vi "Create Generic IO Profile.vi"(8 "error in":errorcluster, 11 "Cia401Profile in":refnum<class "CiA401 Generic IO Profile.lvclass">) -> (0 "error out":errorcluster, 3 "Cia401Profile out":refnum<class "CiA401 Generic IO Profile.lvclass">)   [LabVIEW 2020, in "CiA401 Generic IO Profile.lvclass"]
uses:
  CiA401 Generic IO Profile.lvclass
  CiA401 Generic IO Profile.lvclass/CiA401 Generic IO Profile.ctl
  D:/git/CANopen-LabVIEW/source/Device Profile/Device Profile.lvclass
  D:/git/CANopen-LabVIEW/Profiles/401 Generic IO/CiA401 Generic IO Profile.lvclass
  source/Device Profile/Device Profile.lvclass
  source/Typedefs/Data Type.ctl
  source/CANopen.lvlib
  source/Typedefs/OD Entry Spec.ctl
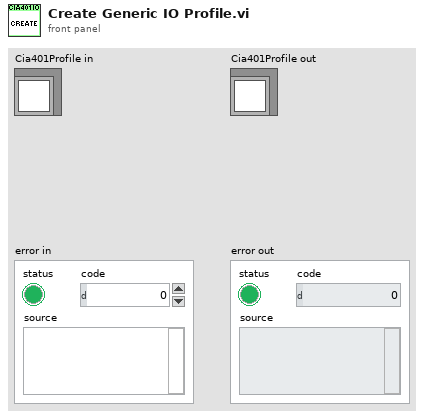
[diagram p1: front panel]
types:
  T1 = typedef "CiA401 Generic IO Profile.lvclass/IO Capabilities.ctl" = cluster{"hasDigitialInputs":bool, "hasDigitalOutputs":bool, "hasAnalogInputs":bool, "hasAnalogOutputs":bool}
  T2 = typedef "CANopen.lvlib/OD Entry Spec.ctl" = cluster{"Index":u16, "Sub Index":u8, "Name":string, "Data Type":T3}
  T3 = typedef "CANopen.lvlib/Data Type.ctl" = u16
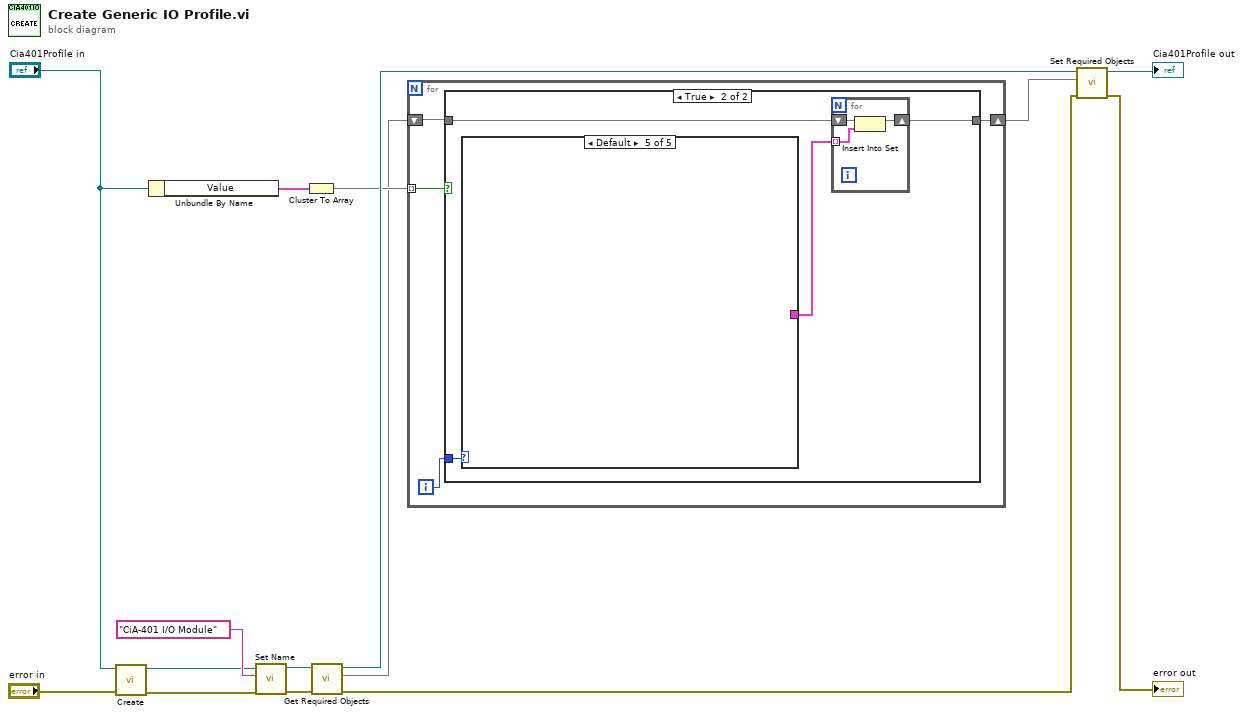
[diagram p0: block diagram]
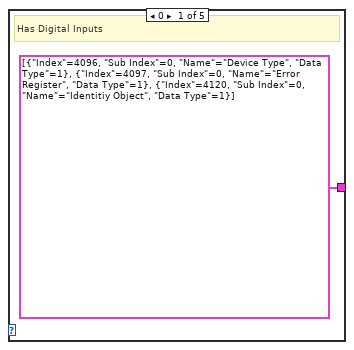
[diagram p3: hidden frame]
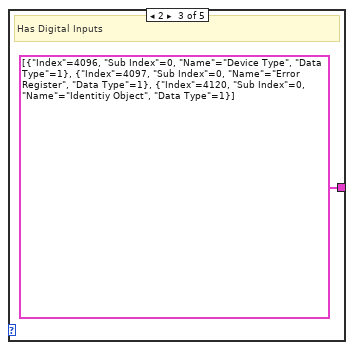
[diagram p5: hidden frame]
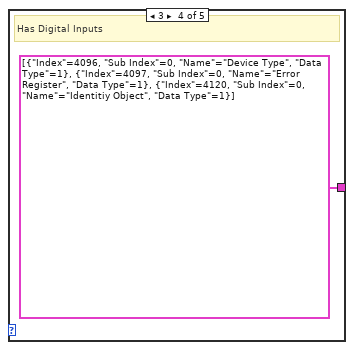
[diagram p6: hidden frame]
diagram:
  n1 = call-dynamic "Create.vi"("error in"="error in", "Device Profile in"="Cia401Profile in") -> ("error out"=w10:errorcluster, "Device Profile out"=w11:refnum<class "CiA401 Generic IO Profile.lvclass">)  [unwired: 8 in]
  n2 = Unbundle By Name("Cia401Profile in") -> ("Value"=w4:T1)
  n3 = call "Set Name.vi"("error in"=w10, "Name"="CiA-401 I/O Module", "Device Profile in"=w11) -> ("error out"=w9:errorcluster, "Device Profile out"=w7:refnum<class "CiA401 Generic IO Profile.lvclass">)  [unwired: 7 in]
  n4 = Cluster To Array(cluster=w4) -> (array=w3:bool[])
  n5 = call "Get Required Objects.vi"("error in"=w9, "Device Profile in"=w7) -> ("error out"=w8:errorcluster, "Required Objects"=w2:set{T2}, "Device Profile out"=w6:refnum<class "CiA401 Generic IO Profile.lvclass">)  [unwired: 7 in]
  n6 = for {
    tunnel: w3 -> [w19] mode=indexing
    shift-right: [w16] -> w1
    shift-left: w2 -> [w17]
    i -> [w18]
    n7 = case shown="True" w19 {
      tunnel: w18 -> [_ w24]
      tunnel: w17 -> [w20 w23]
      tunnel: [w20 w22] -> w16
      frame False {
      }
      frame True {
        n8 = case shown="Default" w24 {
          tunnel: [T2[] [{"Index"=4096, "Sub Index"=0, "Name"="Device Type", "Data Type"=1}, {"Index"=4097, "Sub Index"=0, "Name"="Error Register", "Data Type"=1}, {"Index"=4120, "Sub Index"=0, "Name"="Identitiy Object", "Data Type"=1}] _ T2[] [{"Index"=4096, "Sub Index"=0, "Name"="Device Type", "Data Type"=1}, {"Index"=4097, "Sub Index"=0, "Name"="Error Register", "Data Type"=1}, {"Index"=4120, "Sub Index"=0, "Name"="Identitiy Object", "Data Type"=1}] T2[] [{"Index"=4096, "Sub Index"=0, "Name"="Device Type", "Data Type"=1}, {"Index"=4097, "Sub Index"=0, "Name"="Error Register", "Data Type"=1}, {"Index"=4120, "Sub Index"=0, "Name"="Identitiy Object", "Data Type"=1}] _] -> w21
          frame 0 {
            # "Has Digital Inputs"
          }
          frame 1 {
          }
          frame 2 {
            # "Has Digital Inputs"
          }
          frame 3 {
            # "Has Digital Inputs"
          }
          frame Default {
          }
        }
        n9 = for {
          tunnel: w21 -> [w25] mode=indexing
          shift-right: [w26] -> w22
          shift-left: w23 -> [w27]
          n10 = Insert Into Set(10:w25, 11:w27) -> (3:w26:set{T2})  [unwired: 1 out]
        }
      }
    }
  }
  n11 = call "Set Required Objects.vi"("error in"=w8, "Required Objects"=w1, "Device Profile in"=w6) -> ("error out"=→"error out":errorcluster, "Device Profile out"=→"Cia401Profile out":refnum<class "CiA401 Generic IO Profile.lvclass">)  [unwired: 7 in]
